vi "GaussianFitting.vi"(1 "std":sgl[](array[numeric])=[1.0, 0.0, 5.0], 2 "steps":i32=100, 3 "数组":u16[][](array[numeric])) -> (0 "Result":T1)   [LabVIEW 2012]
uses:
  lib/lm_cpu.dll
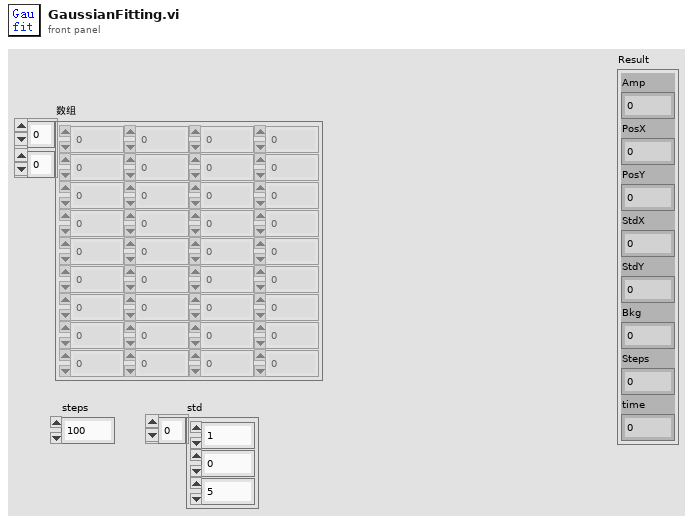
[diagram p1: front panel]
types:
  T1 = cluster{"Amp":dbl, "PosX":dbl, "PosY":dbl, "StdX":dbl, "StdY":dbl, "Bkg":dbl, "Steps":i32, "time":dbl}
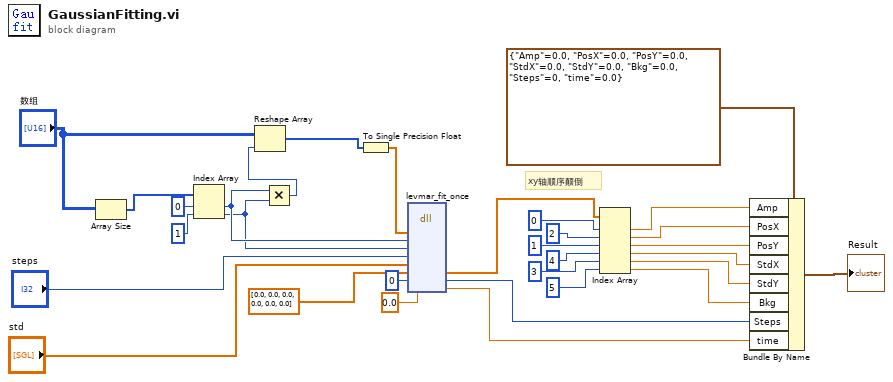
[diagram p0: block diagram]
diagram:
  # "xy轴顺序颠倒"
  n1 = Array Size(array="数组") -> (size(s)=w31:i32[])
  n2 = Index Array(array=w31, index #1=0 ("索引"), index #2=1 ("索引")) -> (element #1=w28:i32, element #2=w20:i32)
  n3 = Multiply(x=w28, y=w20) -> (x*y=w27:i32)
  n4 = Reshape Array("数组", w27) -> (w2:u16[])
  n5 = To Single Precision Float(number=w2) -> (single precision float=w1:sgl[])
  n6 = dll-call lib="D:/github/LVsolis/lib/lm_cpu.dll" fn="levmar_fit_once"("imgedata"=w1, "rows"=w28, "cols"=w20, "steps"="steps", "std"="std", "parsResult"=sgl[] [0.0, 0.0, 0.0, 0.0, 0.0, 0.0], "stepResult"=u32 0, "time"=sgl 0.0) -> ("parsResult"=w13:sgl[], "stepResult"=w5:u32, "time"=w4:sgl)  [unwired: 9 in, 2 out]
  n7 = Index Array(array=w13, index #1=0 ("索引"), index #2=2 ("索引"), index #3=1 ("索引"), index #4=4 ("索引"), index #5=3 ("索引"), index #6=5 ("索引")) -> (element #1=w11:sgl, element #2=w10:sgl, element #3=w9:sgl, element #4=w8:sgl, element #5=w7:sgl, element #6=w6:sgl)
  n8 = Bundle By Name(cluster=T1 {"Amp"=0.0, "PosX"=0.0, "PosY"=0.0, "StdX"=0.0, "StdY"=0.0, "Bkg"=0.0, "Steps"=0, "time"=0.0}, "Amp"=w11, "PosX"=w10, "PosY"=w9, "StdX"=w8, "StdY"=w7, "Bkg"=w6, "Steps"=w5, "time"=w4) -> (→"Result":T1)
